vi "Run Tests in UI.vi"(8 "error in (no error)":errorcluster, 11 "Path":path) -> (0 "error out":errorcluster)   [LabVIEW 2020, in "LUnit Project Provider.lvlib"]
uses:
  LUnit Project Provider.lvlib
  Framework/Execution UI/Public/Execution Mode.ctl
  Framework/Execution UI/Execution UI.lvclass
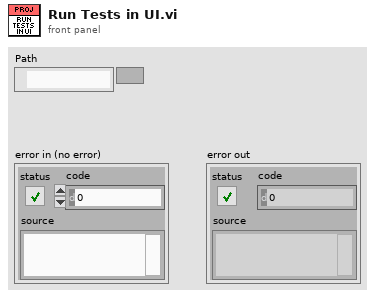
[diagram p1: front panel]
types:
  T1 = enum32{"Invalid", "Standard", "Closed", "Hidden", "Minimized", "Maximized"}
  T2 = typedef "Execution UI.lvclass/Execution Mode.ctl" = enum16{"Default", "Run Tests In Project", "Run Test Case"}
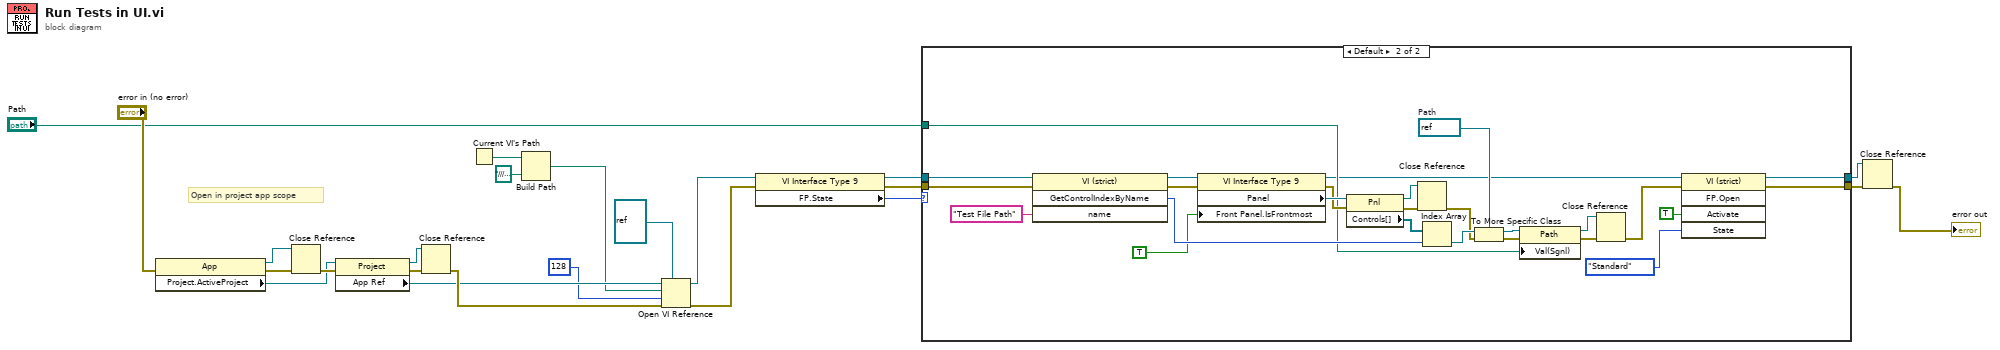
[diagram p0: block diagram]
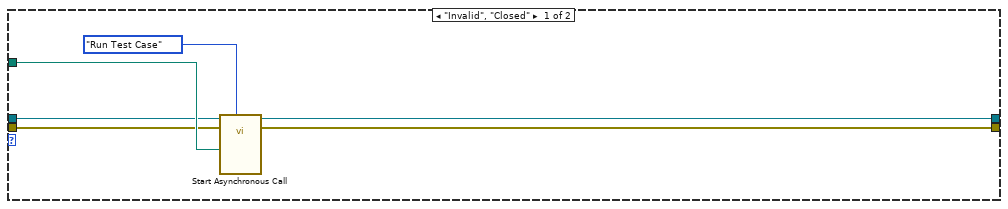
[diagram p2: hidden frame]
diagram:
  # "Open in project app scope"
  n1 = property class="App"(error in="error in (no error)") -> (reference out=w17:refnum<vi>, error out=w15:errorcluster, "Project.ActiveProject"=w10:refnum<vi>)  [unwired: 1 in]
  n2 = Close Reference(reference=w17, error in (no error)=w15) -> (error out=w16:errorcluster)
  n3 = property class="Project"(reference=w10, error in=w16) -> (reference out=w11:refnum<vi>, error out=w13:errorcluster, "App Ref"=w12:refnum<vi>)
  n4 = Close Reference(reference=w11, error in (no error)=w13) -> (error out=w14:errorcluster)
  n5 = Current VI's Path() -> (path=w9:path)
  n6 = Build Path(base path=w9, name or relative path=path "../../../../../vi.lib/Astemes/LUnit/LUnit User Interface.vi" ("Relative Path from 1 to 2")) -> (appended path=w4:path)
  n7 = Open VI Reference(type specifier VI Refnum (for type only)=refnum<vi> refnum, application reference (local)=w12, vi path=w4, options=128, error in (no error)=w14) -> (vi reference=w5:refnum<vi>, error out=w20:errorcluster)  [unwired: 1 in]
  n8 = property class="VI Interface Type 9"(reference=w5, error in=w20) -> (reference out=w18:refnum<vi>, error out=w19:errorcluster, "FP.State"=w21:T1)
  n9 = case shown="Default" w21 {
    tunnel: [w29 w34] -> w1
    tunnel: "Path" -> [w28 w41]
    tunnel: [w26 w35] -> w3
    tunnel: w18 -> [w25 w43]
    tunnel: w19 -> [w24 w42]
    frame "Invalid", "Closed" {
      n10 = call-by-ref "Start Asynchronous Call"(reference=w25, error in=w24, "Execution Mode"=Execution_Mode."Run Test Case", "Test File Path"=w28) -> (reference out=w26:refnum<vi>, error out=w29:errorcluster)  [unwired: 10 in]
    }
    frame Default {
      w50 = refnum<vi> refnum  # Path
      n11 = invoke class="VI (strict)" method="GetControlIndexByName"(reference=w43, error in=w42, "name"="Test File Path" ("Control Name")) -> (reference out=w54:refnum<vi>, error out=w44:errorcluster, "GetControlIndexByName"=w51:i32)  [unwired: 1 in, 1 out]
      n12 = property class="VI Interface Type 9"(reference=w54, error in=w44, "Front Panel.IsFrontmost"=TRUE ("Front Panel Window:Is Frontmost")) -> (reference out=w36:refnum<vi>, error out=w45:errorcluster, "Panel"=w55:refnum<vi>)
      n13 = property class="Pnl"(reference=w55, error in=w45) -> (reference out=w38:refnum<vi>, error out=w46:errorcluster, "Controls[]"=w52:refnum<vi>[])
      n14 = Close Reference(reference=w38, error in (no error)=w46) -> (error out=w39:errorcluster)
      n15 = Index Array(array=w52, index=w51) -> (element=w48:refnum<vi>)
      n16 = To More Specific Class(target class=w50, reference=w48, error in=w39) -> (specific class reference=w49:refnum<vi>, error out=w47:errorcluster)
      n17 = property class="Path"(reference=w49, error in=w47, "Val(Sgnl)"=w41) -> (reference out=w37:refnum<vi>, error out=w40:errorcluster)
      n18 = Close Reference(reference=w37, error in (no error)=w40) -> (error out=w33:errorcluster)
      n19 = invoke class="VI (strict)" method="FP.Open"(reference=w36, error in=w33, "Activate"=TRUE ("Activate?"), "State"=T1."Standard") -> (reference out=w35:refnum<vi>, error out=w34:errorcluster)  [unwired: 1 in, 3 out]
    }
  }
  n20 = Close Reference(reference=w3, error in (no error)=w1) -> (error out=→"error out":errorcluster)
